vi "PXI-4132 Main Page.vi"(8 "error in (no error)":errorcluster, 11 "Node Ptr":T1 format="%.0x") -> (0 "error out":errorcluster)   [LabVIEW 2013, in "PXI-4132 Custom Device.lvlib"]
uses:
  PXI-4132 Custom Device.lvlib
  <vilib>/NI Veristand/Custom Device API/Custom Device Item Ref.ctl
  PXI-4132 Global Variable.vi
  <vilib>/NI Veristand/Custom Device API/Get Item Property (String).vi
  <vilib>/NI Veristand/Custom Device API/Get Item Property (I32).vi
  <vilib>/NI Veristand/Custom Device API/Set Item Property (I32).vi
  <vilib>/NI Veristand/Custom Device API/Set Item Property (String).vi
  <vilib>/NI VeriStand/Custom Device API/Custom Device API.lvlib
panel:
  in  "Hardware Device Name":string
  in  "CPU Assignment":i32
  in  "Decimation":i32
  in  "Header":cluster{"Section Name":string}={"Section Name"="PXI-4132 Settings"}
  in  "Description":string
  in  "Name":string
  # "(-2 is Automatic)"
  # "Hardware Settings"
  # "(Hardware name in MAX)"
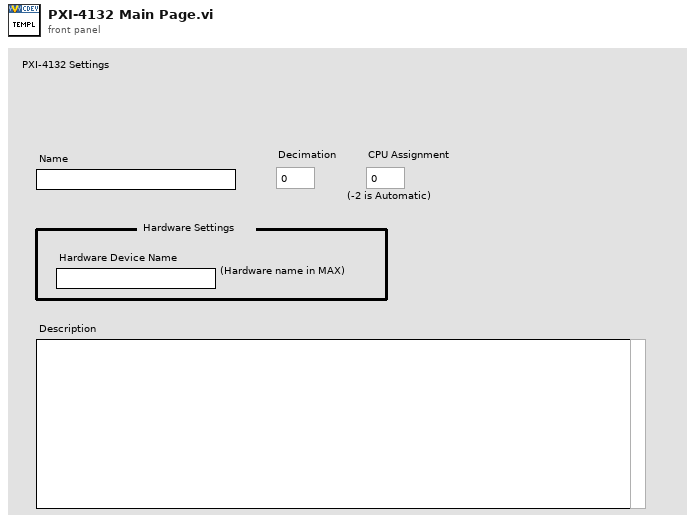
[diagram p1: front panel]
types:
  T1 = typedef "Custom Device API.lvlib/Custom Device Item Ref.ctl" = u64
  T2 = typedef "Custom Device API.lvlib/Custom Device Item Info.ctl" = cluster{"Name":string, "Is Channel":bool, "GUID":string, "Is Waveform":bool}
  T3 = typedef "Custom Device API.lvlib/Custom Device Commands.ctl" = enum16{"Default", "Item renamed", "Shutdown", "Dynamic button pressed"}
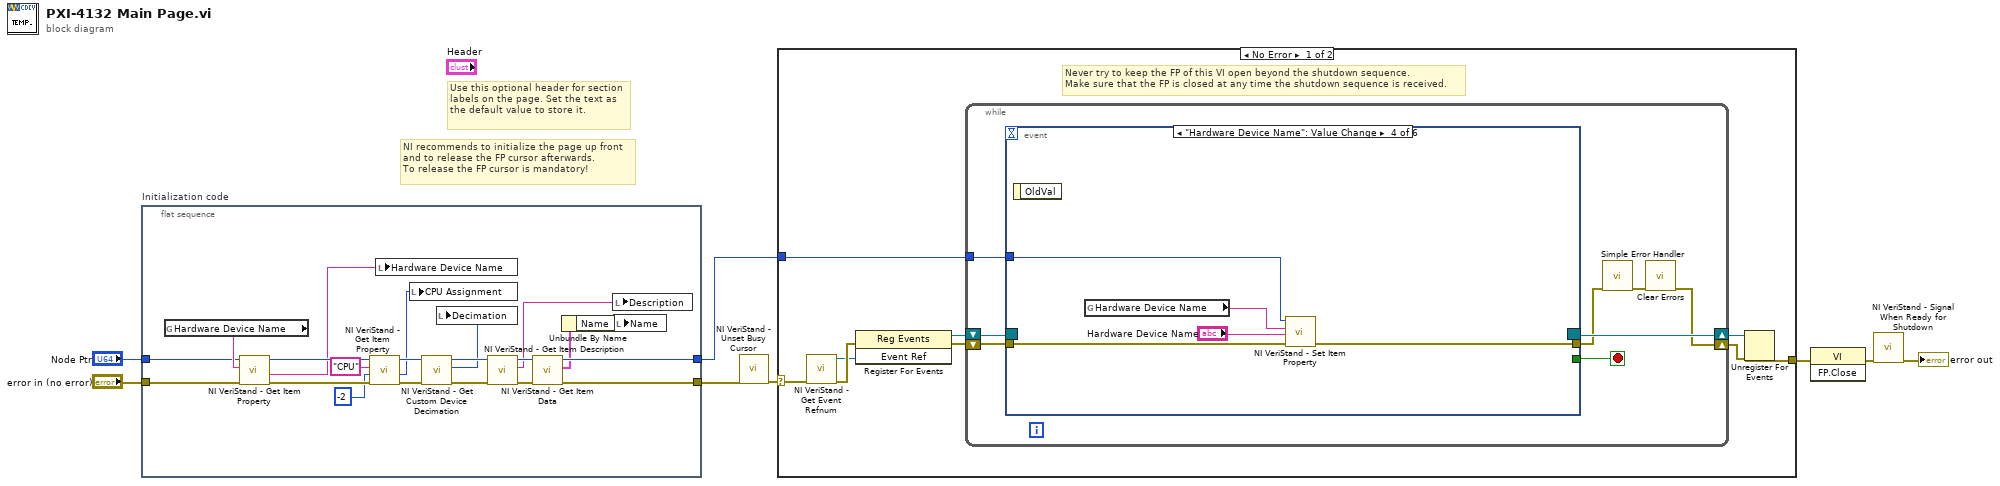
[diagram p0: block diagram]
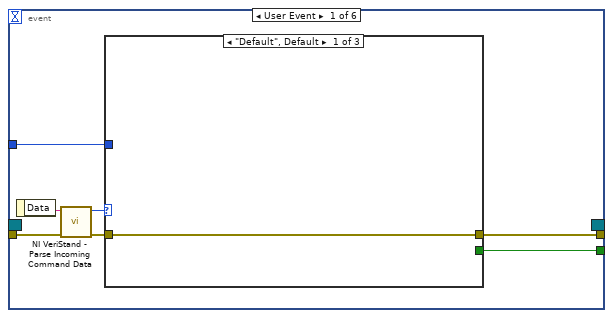
[diagram p2: hidden frame]
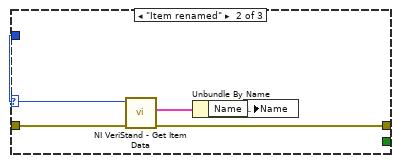
[diagram p3: hidden frame]
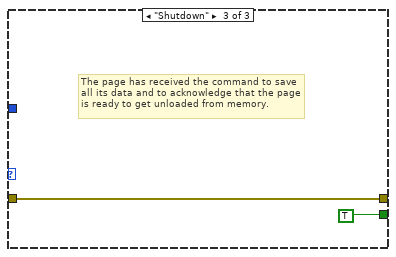
[diagram p4: hidden frame]
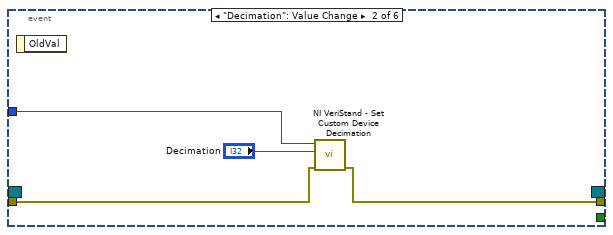
[diagram p5: hidden frame]
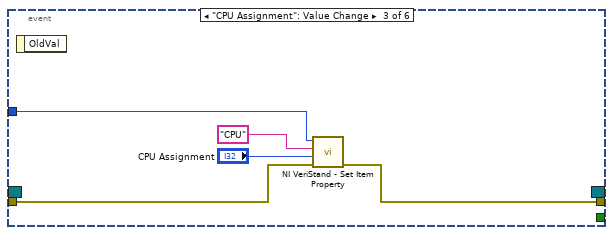
[diagram p6: hidden frame]
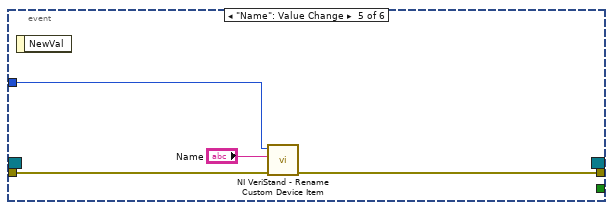
[diagram p7: hidden frame]
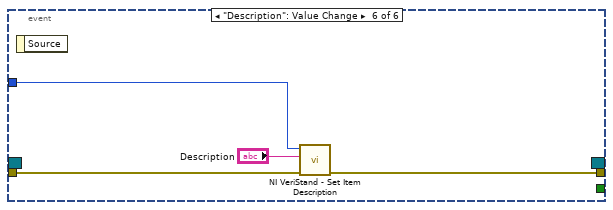
[diagram p8: hidden frame]
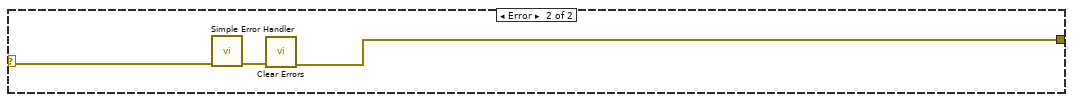
[diagram p9: hidden frame]
diagram:
  # "Use this optional header for section labels on the page. Set the text as the default value to store it."
  # "NI recommends to initialize the page up front\nand to release the FP cursor afterwards.\nTo release the FP cursor is mandatory!"
  n1 = flat-sequence "Initialization code" {
    tunnel: "error in (no error)" -> [w9]
    tunnel: "Node Ptr" -> [w10]
    tunnel: [w23] -> w1
    tunnel: [w29] -> w2
    frame #0 {
      n2 = global read "PXI-4132 Global Variable.vi" "Hardware Device Name"() -> (w15:string)
      n3 = call-poly <vilib>:"NI VeriStand - Get Item Property.vi"("error in (no error)"=w9, "Property Name"=w15, "Item Ref in"=w10) -> ("error out"=w14:errorcluster, "Value"=w12:string, "Item Ref out"=w13:T1)  [unwired: 5 in, 1 out]
      n4 = call-poly <vilib>:"NI VeriStand - Get Item Property.vi"("error in (no error)"=w14, "Default Value"=-2, "Property Name"="CPU", "Item Ref in"=w13) -> ("error out"=w19:errorcluster, "Value"=w17:i32, "Item Ref out"=w21:T1)  [unwired: 4 in, 1 out]
      n5 = local write "Hardware Device Name"(w12) -> ()
      n6 = local write "CPU Assignment"(w17) -> ()
      n7 = call <vilib>:"NI VeriStand - Get Custom Device Decimation.vi"("error in (no error)"=w19, "Device Ref in"=w21) -> ("error out"=w18:errorcluster, "Decimation"=w16:i32, "Device Ref out"=w20:T1)  [unwired: 7 in]
      n8 = local write "Decimation"(w16) -> ()
      n9 = call <vilib>:"NI VeriStand - Get Item Description.vi"("error in (no error)"=w18, "Item Ref in"=w20) -> ("error out"=w26:errorcluster, "Description"=w27:string, "Item Ref out"=w28:T1)  [unwired: 7 out]
      n10 = call <vilib>:"NI VeriStand - Get Item Data.vi"("error in (no error)"=w26, "Item Ref in"=w28) -> ("error out"=w23:errorcluster, "Item Info"=w25:T2, "Item Ref out"=w29:T1)  [unwired: 7 out]
      n11 = Unbundle By Name(w25) -> ("Name"=w24:string)
      n12 = local write "Description"(w27) -> ()
      n13 = local write "Name"(w24) -> ()
    }
  }
  n14 = call <vilib>:"NI VeriStand - Unset Busy Cursor.vi"("error in (no error)"=w1) -> ("error out"=w4:errorcluster)  [unwired: 10 out]
  n15 = case shown="No Error" w4 {
    selector: w4 -> [w30 w86]
    tunnel: [w35 w84] -> w8
    tunnel: w2 -> [w31 _]
    frame No Error {
      # "Never try to keep the FP of this VI open beyond the shutdown sequence.\nMake sure that the FP is closed at any time the shutdown sequence is received."
      n16 = call <vilib>:"NI VeriStand - Get Event Refnum.vi"("error in (no error)"=w30) -> ("error out"=w38:errorcluster, "Event Ref"=w34:refnum<user-event>)  [unwired: 9 out]
      n17 = register-events(error in=w38, w34) -> (reference out=w32:refnum<event-registration>, error out=w33:errorcluster)  [unwired: 1 in]
      n18 = while {
        tunnel: w31 -> [w42]
        shift-right: [w39] -> w36
        shift-left: w33 -> [w45]
        shift-right: [w46] -> w37
        shift-left: w32 -> [w44]
        stop <- w43 stop-if-true
        n19 = event shown="[3] \"Hardware Device Name\": Value Change" {
          selector: w44 -> [_ _ _ _ _ _]
          dyn-events: [_ _ _ _ _ _] -> w46
          timeout: _ -> [_ _ _ _ _ _]
          tunnel: w45 -> [w53 w63 w68 w74 w79 w82]
          tunnel: [w49 _ _ _ _ _] -> w43
          tunnel: [w48 w62 w67 w75 w78 w81] -> w41
          tunnel: w42 -> [w47 w64 w69 w73 w77 w83]
          event User Event {
            n20 = event-data() -> ("Data"=w52:string)  [unwired: 1 out]
            n21 = call <vilib>:"NI VeriStand - Parse Incoming Command Data.vi"("error in (no error)"=w53, "Incoming data"=w52) -> ("error out"=w51:errorcluster, "Action"=w50:T3)  [unwired: 8 out]
            n22 = case shown="\"Default\", Default" w50 {
              tunnel: w51 -> [w54 w59 w60]
              tunnel: [_ _ TRUE] -> w49
              tunnel: [w54 w56 w60] -> w48
              tunnel: w47 -> [_ w58 _]
              frame "Default", Default {
              }
              frame "Item renamed" {
                n23 = call <vilib>:"NI VeriStand - Get Item Data.vi"("error in (no error)"=w59, "Item Ref in"=w58) -> ("error out"=w56:errorcluster, "Item Info"=w57:T2)  [unwired: 8 out]
                n24 = Unbundle By Name(w57) -> ("Name"=w55:string)
                n25 = local write "Name"(w55) -> ()
              }
              frame "Shutdown" {
                # "The page has received the command to save all its data and to acknowledge that the page is ready to get unloaded from memory."
              }
            }
          }
          event "Decimation": Value Change {
            n26 = event-data() -> ()  [unwired: 2 out]
            n27 = call <vilib>:"NI VeriStand - Set Custom Device Decimation.vi"("error in (no error)"=w63, "Decimation"="Decimation", "Device Ref in"=w64) -> ("error out"=w62:errorcluster)  [unwired: 7 in, 1 out]
          }
          event "CPU Assignment": Value Change {
            n28 = event-data() -> ()  [unwired: 2 out]
            n29 = call-poly <vilib>:"NI VeriStand - Set Item Property.vi"("error in (no error)"=w68, "Value"="CPU Assignment", "Property Name"="CPU", "Item Ref in"=w69) -> ("error out"=w67:errorcluster)  [unwired: 5 in, 2 out]
          }
          event "Hardware Device Name": Value Change {
            n30 = event-data() -> ()  [unwired: 2 out]
            n31 = global read "PXI-4132 Global Variable.vi" "Hardware Device Name"() -> (w71:string)
            n32 = call-poly <vilib>:"NI VeriStand - Set Item Property.vi"("error in (no error)"=w74, "Value"="Hardware Device Name", "Property Name"=w71, "Item Ref in"=w73) -> ("error out"=w75:errorcluster)  [unwired: 5 in, 2 out]
          }
          event "Name": Value Change {
            n33 = event-data() -> ()  [unwired: 2 out]
            n34 = call <vilib>:"NI VeriStand - Rename Custom Device Item.vi"("error in (no error)"=w79, "New Name"="Name", "Item Ref in"=w77) -> ("error out"=w78:errorcluster)  [unwired: 1 in, 7 out]
          }
          event "Description": Value Change {
            n35 = event-data() -> ()  [unwired: 2 out]
            n36 = call <vilib>:"NI VeriStand - Set Item Description.vi"("error in (no error)"=w82, "Description"="Description", "Item Ref in"=w83) -> ("error out"=w81:errorcluster)  [unwired: 8 out]
          }
        }
        n37 = call <vilib>:"Simple Error Handler.vi"("error in (no error)"=w41) -> ("error out"=w40:errorcluster)  [unwired: 1 in, 7 out]
        n38 = call <vilib>:"Clear Errors.vi"("error in (no error)"=w40) -> ("error out"=w39:errorcluster)  [unwired: 6 out]
      }
      n39 = Unregister For Events(event registration refnum=w37, error in=w36) -> (error out=w35:errorcluster)
    }
    frame Error {
      n40 = call <vilib>:"Simple Error Handler.vi"("error in (no error)"=w86) -> ("error out"=w85:errorcluster)  [unwired: 1 in, 7 out]
      n41 = call <vilib>:"Clear Errors.vi"("error in (no error)"=w85) -> ("error out"=w84:errorcluster)  [unwired: 6 out]
    }
  }
  n42 = invoke class="VI" method="FP.Close"(error in=w8) -> (error out=w7:errorcluster)  [unwired: 2 in, 2 out]
  n43 = call <vilib>:"NI VeriStand - Signal When Ready for Shutdown.vi"("error in (no error)"=w7) -> ("error out"=→"error out":errorcluster)  [unwired: 10 out]
